vi "Self Msg Send.vi"(9 "Priority Msg?":bool, 10 "Msg":refnum<class "Msg Strategy.lvclass">, 11 "Msg Sends in":refnum<class "Msg Sends.lvclass">) -> (0 "error out":errorcluster)   [LabVIEW 2021, in "LVCAM.lvlib" / "Msg Sends.lvclass"]
uses:
  Msg Sends.lvclass
  Msg Strategy/Msg Strategy.lvclass
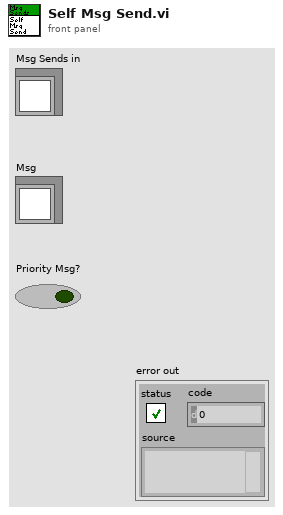
[diagram p1: front panel]
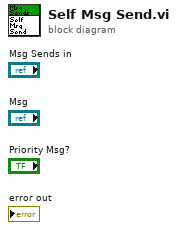
[diagram p0: block diagram]
diagram:
